vi "Is Trigger Mode Available.vi"(8 "error in (no error)":errorcluster, 11 "iTriggerMode":i32) -> (0 "error out":errorcluster, 3 "function return":u32)   [LabVIEW 2014, in "atmcd32d.lvlib"]
doc: "unsigned int WINAPI IsTriggerModeAvailable(int iTriggerMode);"
uses:
  atmcd32d.lvlib
  atmcd32d.dll
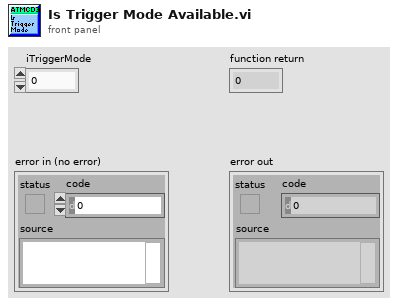
[diagram p1: front panel]
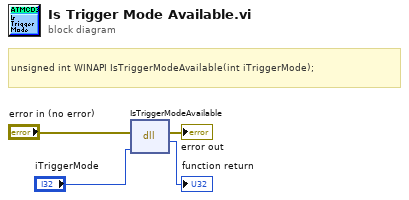
[diagram p0: block diagram]
diagram:
  # "unsigned int WINAPI IsTriggerModeAvailable(int iTriggerMode);"
  n1 = dll-call lib="C:/Users/Bakir/Documents/Lambda2-Testing/lib/Andorlib/atmcd32d.*" fn="IsTriggerModeAvailable"(error in="error in (no error)", "iTriggerMode"="iTriggerMode") -> (error out=→"error out":errorcluster, →"function return":u32)  [unwired: 3 in, 1 out]
